vi "Get Reservable Resources.vi"(8 "error in (no error)":errorcluster, 11 "CD Ref in":T1 format="%.0x") -> (0 "error out":errorcluster, 2 "Reservable Resources":T2[](array[typedef]) {"fpga cd" format="%.0x"}, 3 "CD Ref out":T1 format="%.0x")   [LabVIEW 2016, in "FPGA RM System Definition API.lvlib"]
uses:
  FPGA RM System Definition API.lvlib
  <vilib>/NI Veristand/Custom Device API/Custom Device Item Ref.ctl
  Types/resources.ctl
  Types/fpga resource.ctl
  Types/Channel Type.ctl
  <vilib>/NI VeriStand/Custom Device API/Custom Device API.lvlib
  Shared/FPGA RM Shared API.lvlib
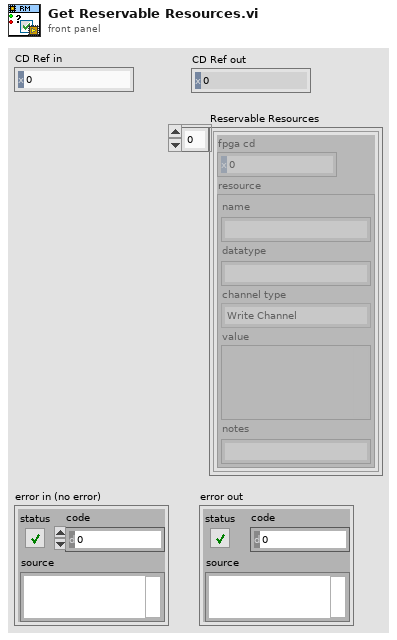
[diagram p1: front panel]
types:
  T1 = typedef "Custom Device API.lvlib/Custom Device Item Ref.ctl" = u64
  T2 = typedef "FPGA RM System Definition API.lvlib/resources.ctl" = cluster{"fpga cd":T1, "resource":T3}
  T3 = typedef "FPGA RM Shared API.lvlib/fpga resource.ctl" = cluster{"name":string, "datatype":string, "channel type":T4, "value":variant, "notes":string}
  T4 = typedef "FPGA RM Shared API.lvlib/Channel Type.ctl" = enum16{"Write Channel", "Read Channel", "Write Waveform", "Read Waveform"}
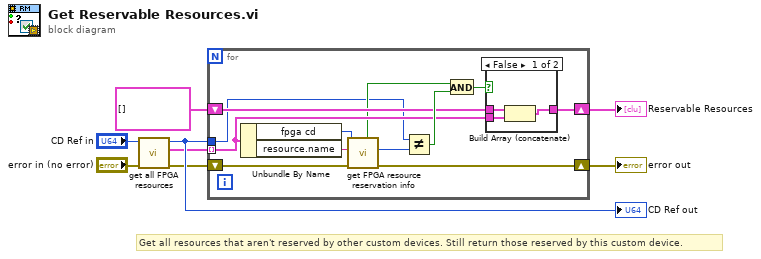
[diagram p0: block diagram]
diagram:
  # "Get all resources that aren't reserved by other custom devices. Still return those reserved by this custom device."
  n1 = call "get all FPGA resources.vi"("error in (no error)"="error in (no error)", "Item Ref in"="CD Ref in") -> ("error out"=w4:errorcluster, "fpga resources"=w5:T2[], "Item Ref out"=w8:T1)  [unwired: 7 in]
  "CD Ref out" <- w8
  n2 = for {
    tunnel: w5 -> [w12] mode=indexing
    shift-right: [w16] -> w6
    shift-left: w4 -> [w20]
    shift-right: [w14] -> w7
    shift-left: T2[] [] ("fpga resources") -> [w13]
    tunnel: w8 -> [w9]
    n3 = Unbundle By Name(w12) -> ("fpga cd"=w10:T1, "resource.name"=w19:string)
    n4 = call "get FPGA resource reservation info.vi"("error in (no error)"=w20, "Name in Bitfile"=w19, "Item Ref in"=w10) -> ("error out"=w16:errorcluster, "Reserver Node Ref"=w18:T1, "reserved?"=w11:bool)  [unwired: 3 in, 3 out]
    n5 = Not Equal?(x=w9, y=w18) -> (x != y?=w17:bool)
    n6 = And(x=w11, y=w17) -> (x .and. y?=w15:bool)
    n7 = case shown="False" w15 {
      tunnel: w12 -> [w23 _]
      tunnel: [w22 w24] -> w14
      tunnel: w13 -> [w21 w24]
      frame False {
        n8 = Build Array (concatenate)(w21, w23) -> (w22:T2[])
      }
      frame True {
      }
    }
  }
  "Reservable Resources" <- w7
  "error out" <- w6
